vi "ConnectErrorCodes.vi"() -> (4 "[user-defined codes]":i32[](array[numeric])=[0, -1, -3, -4, -5, -7, -9], 8 "[user-defined descriptions]":string[](array[string])=["no error", "function error", "invalid serial port (port is not found)", "access denied  (port is busy)", "no response from control unit", "control unit with the specified serial number is not found", "no connection to tcp/ip socket"])   [LabVIEW 2020]
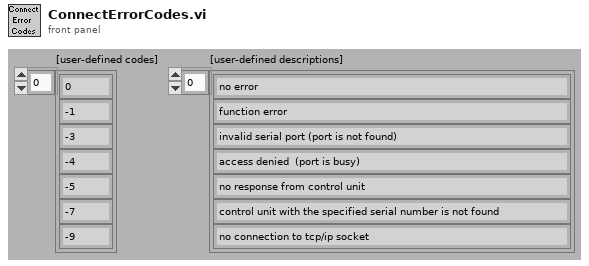
[diagram p1: front panel]
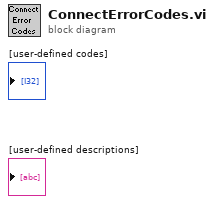
[diagram p0: block diagram]
diagram:
